vi "create_csv.vi"(8 "error in":errorcluster, 10 "CSV name":string, 11 "ship path":path) -> (0 "error out":errorcluster, 3 "csv path":path)   [LabVIEW 2020]
uses:
  <vilib>/regexp/Match Regular Expression.xnode
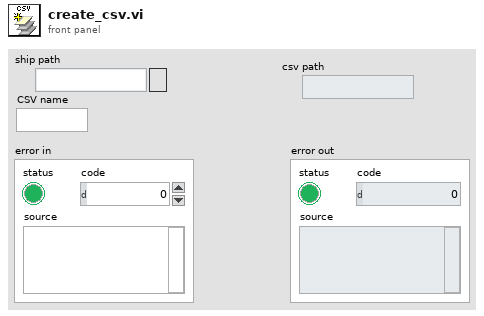
[diagram p1: front panel]
types:
  T1 = enum16{"open", "replace", "create", "open or create", "replace or create", "replace or create with confirmation"}
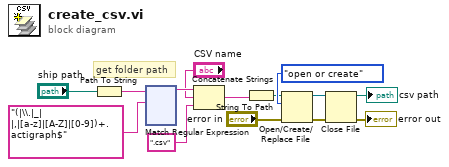
[diagram p0: block diagram]
diagram:
  # "get folder path"
  n1 = Path To String(path="ship path") -> (string=w8:string)
  n2 = xnode "Match Regular Expression"("input string"=w8, "regular expression"="(|\\.|_| |,|[a-z]|[A-Z]|[0-9])+.actigraph$") -> ("before match"=w9:string)  [unwired: 4 in, 4 out]
  n3 = Concatenate Strings(w9, "CSV name", ".csv" ("extension")) -> (w5:string)
  n4 = String To Path(string=w5) -> (path=w13:path)
  n5 = Open/Create/Replace File(file path (use dialog)=w13, error in="error in", operation (0:open)=T1."open or create") -> (refnum out=w11:refnum<file>, error out=w12:errorcluster)  [unwired: 3 in, 1 out]
  n6 = Close File(refnum=w11, error in=w12) -> (path=→"csv path":path, error out=→"error out":errorcluster)
